vi "Refresh Z Scale Positions.vi"(8 "Z Scale Refs":refnum<vi>[](array[refnum]), 11 "IMAQ Display Refs":refnum<vi>[](array[refnum])) -> ()   [LabVIEW 2016]
uses:
  <vilib>/Utility/miscctls.llb/LVPositionTypeDef.ctl
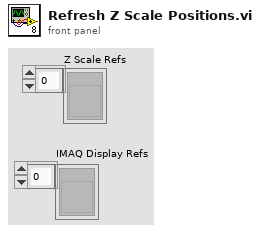
[diagram p1: front panel]
types:
  T1 = typedef "LVPositionTypeDef.ctl" = cluster{"Left":i32, "Top":i32}
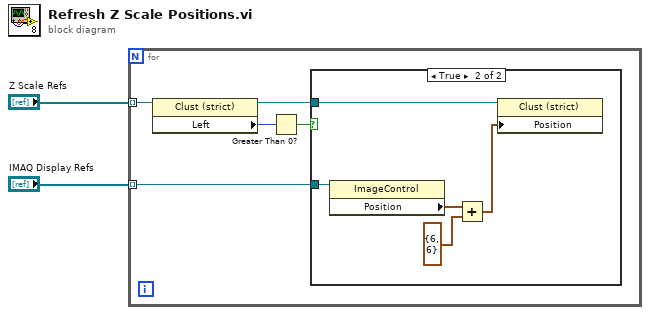
[diagram p0: block diagram]
diagram:
  n1 = for {
    tunnel: "Z Scale Refs" -> [w7] mode=indexing
    tunnel: "IMAQ Display Refs" -> [w3] mode=indexing
    n2 = property class="Clust (strict)"(reference=w7) -> (reference out=w4:refnum<vi>, "Left"=w6:i32)  [unwired: 1 in, 1 out]
    n3 = Greater Than 0?(x=w6) -> (x > 0?=w5:bool)
    n4 = case shown="True" w5 {
      tunnel: w4 -> [_ w9]
      tunnel: w3 -> [_ w12]
      frame False {
      }
      frame True {
        n5 = property class="ImageControl"(reference=w12) -> ("Position"=w11:T1)  [unwired: 1 in, 2 out]
        n6 = Add(x=w11, y=T1 {"Left"=6, "Top"=6}) -> (x+y=w8:T1)
        n7 = property class="Clust (strict)"(reference=w9, "Position"=w8) -> ()  [unwired: 1 in, 2 out]
      }
    }
  }
